vi "Get all Targets.vi"(8 "error in":errorcluster, 11 "Project Selection":string) -> (0 "error out":errorcluster, 3 "Targets":string[](array[string]))   [LabVIEW 2019, in "Panther Dashboard.lvlib"]
uses:
  Panther Dashboard.lvlib
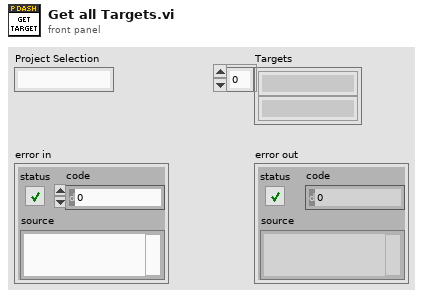
[diagram p1: front panel]
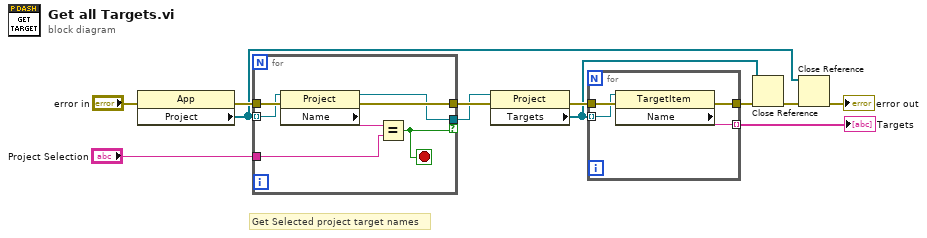
[diagram p0: block diagram]
diagram:
  # "Get Selected project target names"
  n1 = property class="App"(error in="error in") -> (error out=w10:errorcluster, "Project"=w3:refnum<vi>[])  [unwired: 1 in, 1 out]
  n2 = for {
    tunnel: w3 -> [w17] mode=indexing
    tunnel: [w14] -> w6 if=w13
    tunnel: "Project Selection" -> [w15]
    tunnel: w10 -> [w19]
    tunnel: [w18] -> w9
    stop <- w13 stop-if-true
    n3 = property class="Project"(reference=w17, error in=w19) -> (reference out=w14:refnum<vi>, error out=w18:errorcluster, "Name"=w16:string)
    n4 = Equal?(x=w16, y=w15) -> (x = y?=w13:bool)
  }
  n5 = property class="Project"(reference=w6, error in=w9) -> (error out=w11:errorcluster, "Targets"=w2:refnum<vi>[])  [unwired: 1 out]
  n6 = for {
    tunnel: w2 -> [w21] mode=indexing
    tunnel: [w20] -> w4 mode=indexing
    tunnel: w11 -> [w23]
    tunnel: [w22] -> w1
    n7 = property class="TargetItem"(reference=w21, error in=w23) -> (error out=w22:errorcluster, "Name"=w20:string)  [unwired: 1 out]
  }
  "Targets" <- w4
  n8 = Close Reference(reference=w2, error in (no error)=w1) -> (error out=w7:errorcluster)
  n9 = Close Reference(reference=w3, error in (no error)=w7) -> (error out=→"error out":errorcluster)
